vi "Periodic Tasks.vi"(8 "error in":errorcluster) -> ()   [LabVIEW 2016]
doc: "This VI runs in parallel to other robot code. It can contain as many user-defined periodic loops as you need. These can carry out PID or other sorts of timed response."
uses:
  <vilib>/Rock Robotics/WPI/ThirdParty/CanMotor/TalonSRX/WPI_CANTalonSRX_APIControlMode.ctl
  <vilib>/Rock Robotics/WPI/Utilities/WPI_GetSetVariantRefNum.vi
  Robot Global Data.vi
  <vilib>/Rock Robotics/Network Tables/NT Write Boolean.vi
  <vilib>/Rock Robotics/Network Tables/NT Write Number.vi
  <vilib>/Rock Robotics/Network Tables/NT Write Numeric Array.vi
panel:
  out "R3 Latch Shooter":bool
  out "LIDAR Dist IN":dbl
  out "Shooter Speed Increment":dbl=2000.0 format="%#_13g"
  out "LIDAR Dist CM":u16
  # "Gear Catcher forwards, Encoder 1 = +4096\n  Gear Catcher forwards, Encoder 1 = -4096"
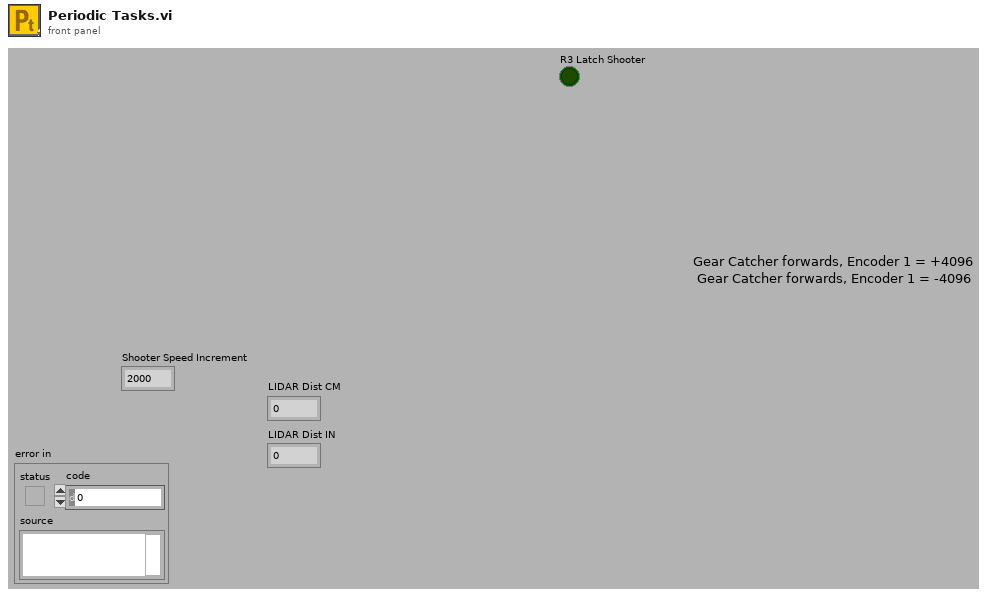
[diagram p1: front panel]
types:
  T1 = typedef "WPI_JoystickDevRef.ctl" = cluster{"Device":T2}
  T2 = typedef "WPI_JoystickDeviceEnum.ctl" = enum16{"USB 0", "USB 1", "USB 2", "USB 3", "USB 4", "USB 5"}
  T3 = typedef "WPI_I2CDevRef.ctl" = cluster{"DevStatus":errorcluster, "Device Address":u8, "Handle":i32, "I2C Bus":T4}
  T4 = typedef "i2c_bus.ctl" = enum16{"I2C On-Board", "I2C MXP", "Invalid"}
  T5 = typedef "WPI_MotorControlDeviceRef.ctl" = cluster{"DeviceStatus":errorcluster, "Type":T6, "PWM":cluster{"PWM Channel":T7, "DeadBand":T8}, "CAN":cluster{"Device Number":u8, "SetOutput VI Ref":variant, "GetOutput VI Ref":variant, "Enable VI Ref":variant, "Disable VI Ref":variant, "Data":variant}, "Invert":bool}
  T6 = typedef "WPI_MotorControlType.ctl" = enum16{"PWM", "CAN"}
  T7 = typedef "FPGA_DIOPWMChannel.ctl" = enum8{"PWM 0", "PWM 1", "PWM 2", "PWM 3", "PWM 4", "PWM 5", "PWM 6", "PWM 7", "PWM 8", "PWM 9", "PWM MXP 0", "PWM MXP 1", "PWM MXP 2", "PWM MXP 3", "PWM MXP 4", "PWM MXP 5", "PWM MXP 6", "PWM MXP 7", "PWM MXP 8", "PWM MXP 9", "Invalid"}
  T8 = typedef "WPI_PWMDeadband.ctl" = cluster{"Name":string, "maxPositivePwm":i32, "minPositivePwm":i32, "centerPwm":i32, "maxNegativePwm":i32, "minNegativePwm":i32, "angularRange":u16}
  T9 = typedef "WPI_CANTalonSRX_APIControlMode.ctl" = enum8{"Percent VBus", "Speed", "Position", "Slave", "Unchanged / Invalid", "Voltage Compensation", "Current", "Motion Profile", "Motion Magic"}
  T10 = typedef "WPI_CANTalonSRX_GlobalStatus.ctl" = cluster{"Applied Throttle":dbl, "Module Enabled":bool, "CAN Error":errorcluster, "Closed Loop Error":dbl, "Forward Limit Switch Closed":bool, "Reverse Limit Switch Closed":bool, "Sensor Position":dbl, "Sensor Velocity":dbl, "Current":dbl, "Sticky Fault - Over Temp":bool, "Sticky Fault - Under Voltage":bool, "Sticky Fault - Forward Limit":bool, "Sticky Fault - Reverse Limit":bool, "Sticky Fault - Forward Soft Limit":bool, "Sticky Fault - Reverse Soft Limit":bool, "Brake is Enabled":bool, "Encoder Position":dbl, "Encoder Velocity":dbl, "Encoder Index Count":dbl, "Encoder A Pin State":bool, "Encoder B Pin State":bool, "Encoder Index Pin State":bool, "Analog In":dbl, "Analog In Velocity":dbl, "Temperature (C)":dbl, "Battery Voltage":dbl, "Control 5 Is Supported":bool, "Current Profile Slot Select":dbl, "Pos Div 8":bool, "Vel Div 4":bool, "Pulse Width Position":i32, "Pulse Width Velocity":i32, "Pulse Width Rise To Rise (us)":i32, "Pulse Width Rise To Fall (us)":i32, "Mot Prof Active Is Under Run":bool, "Mot Prof Active Has Under Run":bool, "Mot Prof Active Is Last":bool, "Mot Prof Active Velocity Only":bool, "Mot Prof Active Is Valid":bool, "Mot Prof Buffer Is Full":bool, "Mot Prof Active Profile Slot Select":i32, "Mot Prof NextID":i32, "Mot Prof Count":i32, "Mot Prof Active Velocity":dbl, "Mot Prof Active Position":dbl, "Mot Prof Output Enable":i32}
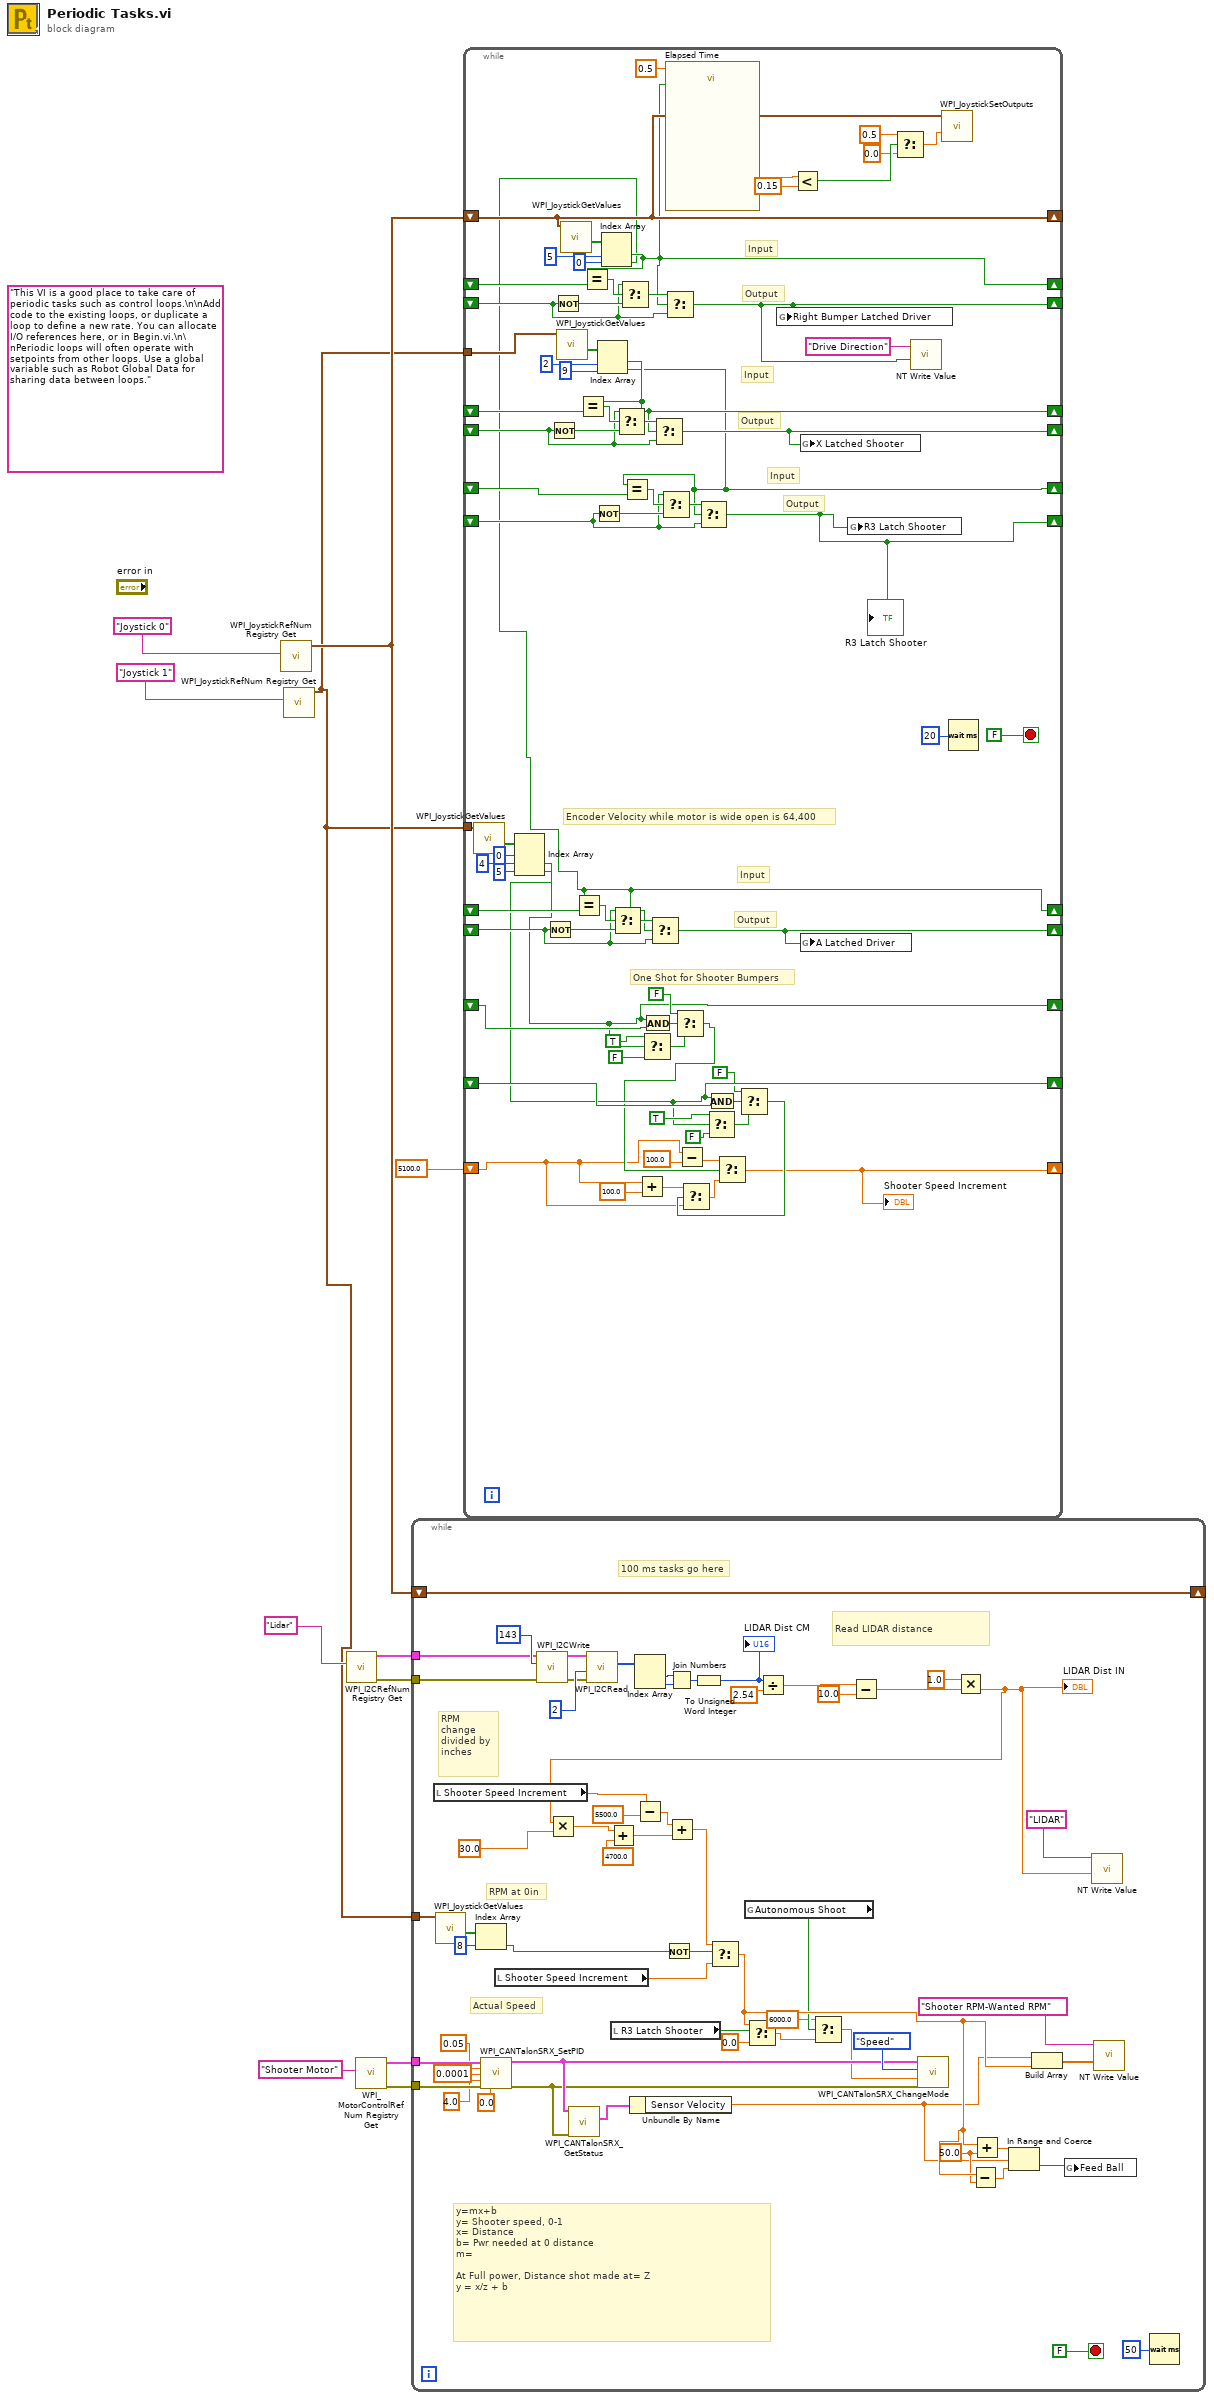
[diagram p0: block diagram]
diagram:
  (unwired) "This VI is a good place to take care of periodic tasks such as control loops.\n\nAdd code to the existing loops, or duplicate a loop to define a new rate. You can allocate I/O references here, or in Begin.vi.\n\nPeriodic loops will often operate with setpoints from other loops. Use a global variable such as Robot Global Data for sharing data between loops."
  n1 = call <vilib>:"WPI_JoystickRefNum Registry Get.vi"("refnum name"="Joystick 0") -> ("JoystickDevRef"=w10:T1)  [unwired: 1 in, 9 out]
  n2 = call <vilib>:"WPI_JoystickRefNum Registry Get.vi"("refnum name"="Joystick 1") -> ("JoystickDevRef"=w1:T1)  [unwired: 1 in, 9 out]
  n3 = call <vilib>:"WPI_I2CRefNum Registry Get.vi"("refnum name"="Lidar") -> ("error out"=w5:errorcluster, "I2CDevRef"=w7:T3)  [unwired: 9 in]
  n4 = call <vilib>:"WPI_MotorControlRefNum Registry Get.vi"("refnum name"="Shooter Motor") -> ("error out"=w2:errorcluster, "MotorControlDevRef"=w3:T5)  [unwired: 9 in]
  n5 = while {
    shift-right: [w68] -> _
    shift-left: w10 -> [w68]
    tunnel: w7 -> [w59]
    tunnel: w5 -> [w55]
    tunnel: w3 -> [w50]
    tunnel: w2 -> [w49]
    tunnel: w1 -> [w13]
    stop <- FALSE stop-if-true
    w32 = 50.0 ("y")
    # "RPM at 0in"
    # "RPM change divided by inches"
    # "y=mx+b\ny= Shooter speed, 0-1\nx= Distance\nb= Pwr needed at 0 distance\nm= \n\nAt Full power, Distance shot made at= Z\ny = x/z + b"
    # "Actual Speed"
    # "Read LIDAR distance"
    # "100 ms tasks go here"
    n6 = local read "Shooter Speed Increment"() -> (w18:dbl)
    n7 = call <vilib>:"WPI_JoystickGetValues.vi"("JoystickDevRef"=w13) -> ("Buttons"=w14:bool[])  [unwired: 6 in, 4 out]
    n8 = Index Array(array=w14, index=8) -> (element=w12:bool)
    n9 = call <vilib>:"WPI_CANTalonSRX_SetPID.vi"("CAN Talon SRX Ref"=w50, "P"=0.05, "I"=0.0001, "D"=4.0, "error in (no error)"=w49, "F"=0.0) -> ("CAN Talon SRX Ref"=w41:T5, "error out"=w40:errorcluster)  [unwired: 8 in]
    n10 = local read "Shooter Speed Increment"() -> (w36:dbl)
    n11 = call <vilib>:"WPI_I2CWrite.vi"("error in (no error)"=w55, "I2CRegister"=u8 143 ("Device Address"), "I2CDevRef"=w59) -> ("error out"=w60:errorcluster, "I2CDevRef"=w61:T3)  [unwired: 7 in]
    n12 = call <vilib>:"WPI_CANTalonSRX_GetStatus.vi"("error in (no error)"=w40, "CAN Talon SRX Ref"=w41) -> ("Talon SRX Status"=w39:T10)  [unwired: 7 in, 2 out]
    n13 = call <vilib>:"WPI_I2CRead.vi"("error in (no error)"=w60, "I2CBytesToRead"=u8 2, "I2CDevRef"=w61) -> ("Data Out"=w67:u8[])  [unwired: 6 in, 2 out]
    n14 = local read "R3 Latch Shooter"() -> (w43:bool)
    n15 = Unbundle By Name(w39) -> ("Sensor Velocity"=w22:dbl)
    n16 = Index Array(array=w67) -> (element #1=w66:u8, element #2=w65:u8)  [unwired: 2 in]
    n17 = Subtract(x=w18, y=5500.0) -> (x-y=w19:dbl)
    n18 = Not(x=w12) -> (.not. x?=w16:bool)
    n19 = Join Numbers(hi=w66, lo=w65) -> ((hi.lo)=w64:u16)
    n20 = To Unsigned Word Integer(number=w64) -> (unsigned 16bit integer=w58:u16)
    "LIDAR Dist CM" <- w58
    n21 = global read "Robot Global Data.vi" "Autonomous Shoot"() -> (w26:bool)
    n22 = Divide(x=w58, y=2.54) -> (x/y=w57:dbl)
    n23 = Subtract(x=w57, y=10.0) -> (x-y=w54:dbl)
    n24 = Multiply(x=1.0, y=w54) -> (x*y=w23:dbl)
    "LIDAR Dist IN" <- w23
    n25 = Multiply(x=w23, y=30.0 ("RPM change/ Inches")) -> (x*y=w30:dbl)
    n26 = Add(x=w30, y=4700.0 ("RPM at 0 in")) -> (x+y=w21:dbl)
    n27 = Add(x=w19, y=w21) -> (x+y=w20:dbl)
    n28 = Select(t=w20, s=w16, f=w36) -> (s? t:f=w33:dbl)
    n29 = Select(t=w33, s=w43, f=0.0) -> (s? t:f=w28:dbl)
    n30 = Select(t=6000.0, s=w26, f=w28) -> (s? t:f=w27:dbl)
    n31 = call <vilib>:"WPI_CANTalonSRX_ChangeMode.vi"("error in (no error)"=w40, "Output"=w27, "Control Mode"=WPI_CANTalonSRX_APIControlMode."Speed", "CAN Talon SRX Ref"=w41) -> ()  [unwired: 6 in, 2 out]
    n32 = Subtract(x=w33, y=w32) -> (x-y=w34:dbl)
    n33 = Add(x=w33, y=w32) -> (x+y=w35:dbl)
    n34 = In Range and Coerce(upper limit=w35, x=w22, lower limit=w34) -> (In Range?=w31:bool)  [unwired: 1 out]
    n35 = Build Array(w22, w33) -> (w38:dbl[])
    n36 = global write "Robot Global Data.vi" "Feed Ball"(w31) -> ()
    n37 = call-poly <vilib>:"NT Write Value.vi"("Numeric"=w23, "Name"="LIDAR") -> ()  [unwired: 9 in, 1 out]
    n38 = call-poly <vilib>:"NT Write Value.vi"("Numeric Array"=w38, "Name"="Shooter RPM-Wanted RPM") -> ()  [unwired: 9 in, 1 out]
    n39 = Wait (ms)(milliseconds to wait=u32 50) -> ()  [unwired: 1 out]
  }
  n40 = while {
    shift-right: [w117] -> _
    shift-left: w10 -> [w117]
    shift-right: [w115] -> _
    shift-left: _ -> [w139]
    shift-right: [w71] -> _
    shift-left: _ -> [w136]
    tunnel: w1 -> [w130]
    shift-right: [w129] -> _
    shift-left: _ -> [w126]
    shift-right: [w128] -> _
    shift-left: _ -> [w127]
    shift-right: [w119] -> _
    shift-left: _ -> [w121]
    shift-right: [w118] -> _
    shift-left: _ -> [w122]
    shift-right: [w73] -> _
    shift-left: _ -> [w105]
    shift-right: [w103] -> _
    shift-left: _ -> [w104]
    tunnel: w1 -> [w100]
    shift-right: [w93] -> _
    shift-left: _ -> [w96]
    shift-right: [w85] -> _
    shift-left: _ -> [w86]
    shift-right: [w77] -> _
    shift-left: 5100.0 -> [w76]
    stop <- FALSE stop-if-true
    # "One Shot for Shooter Bumpers"
    # "Encoder Velocity while motor is wide open is 64,400"
    # "Output"
    # "Input"
    # "Output"
    # "Input"
    # "Output"
    # "Input"
    # "Output"
    # "Input"
    n41 = call <vilib>:"WPI_JoystickGetValues.vi"("JoystickDevRef"=w100) -> ("Buttons"=w101:bool[])  [unwired: 6 in, 4 out]
    n42 = Index Array(array=w101, index #1=0 ("index"), index #2=4 ("index"), index #3=5 ("index")) -> (element #2=w93:bool, element #3=w85:bool)  [unwired: 1 out]
    n43 = Not(x=w104) -> (.not. x?=w106:bool)
    n44 = Not(x=w127) -> (.not. x?=w131:bool)
    n45 = Not(x=w136) -> (.not. x?=w137:bool)
    n46 = call <vilib>:"WPI_JoystickGetValues.vi"("JoystickDevRef"=w130) -> ("Buttons"=w135:bool[])  [unwired: 6 in, 4 out]
    n47 = call <vilib>:"WPI_JoystickGetValues.vi"("JoystickDevRef"=w117) -> ("Buttons"=w142:bool[])  [unwired: 6 in, 4 out]
    n48 = Not(x=w122) -> (.not. x?=w123:bool)
    n49 = Index Array(array=w135, index #1=2 ("index"), index #2=9 ("index")) -> (element #1=w129:bool, element #2=w119:bool)
    n50 = Equal?(x=w129, y=w126) -> (x = y?=w133:bool)
    n51 = Index Array(array=w142, index #1=5 ("index"), index #2=0 ("index")) -> (element #1=w115:bool, element #2=w73:bool)
    n52 = Equal?(x=w73, y=w105) -> (x = y?=w108:bool)
    n53 = Equal?(x=w115, y=w139) -> (x = y?=w140:bool)
    n54 = Select(t=w104, s=w108, f=w106) -> (s? t:f=w107:bool)
    n55 = Select(t=w127, s=w133, f=w131) -> (s? t:f=w132:bool)
    n56 = Select(t=w136, s=w140, f=w137) -> (s? t:f=w138:bool)
    n57 = Equal?(x=w119, y=w121) -> (x = y?=w125:bool)
    n58 = Add(x=w76, y=100.0) -> (x+y=w80:dbl)
    n59 = Select(t=TRUE, s=w93, f=FALSE) -> (s? t:f=w94:bool)
    n60 = And(x=w93, y=w96) -> (x .and. y?=w97:bool)
    n61 = Select(t=w107, s=w73, f=w104) -> (s? t:f=w103:bool)
    n62 = Select(t=w132, s=w129, f=w127) -> (s? t:f=w128:bool)
    n63 = Select(t=w122, s=w125, f=w123) -> (s? t:f=w124:bool)
    n64 = Select(t=w138, s=w115, f=w136) -> (s? t:f=w71:bool)
    n65 = call "Elapsed Time"("Time Target (s)"=0.5, "Reset"=w115) -> ("Elapsed Time (s)"=w114:dbl)  [unwired: 10 in, 7 out]
    n66 = Select(t=FALSE, s=w97, f=w94) -> (s? t:f=w83:bool)
    n67 = Subtract(x=w76, y=100.0 ("x")) -> (x-y=w82:dbl)
    n68 = Select(t=w124, s=w119, f=w122) -> (s? t:f=w118:bool)
    "R3 Latch Shooter" <- w118
    n69 = Select(t=TRUE, s=w85, f=FALSE) -> (s? t:f=w89:bool)
    n70 = And(x=w85, y=w86) -> (x .and. y?=w90:bool)
    n71 = Select(t=FALSE, s=w90, f=w89) -> (s? t:f=w79:bool)
    n72 = Select(t=w80, s=w79, f=w76) -> (s? t:f=w81:dbl)
    n73 = Select(t=w82, s=w83, f=w81) -> (s? t:f=w77:dbl)
    "Shooter Speed Increment" <- w77
    n74 = global write "Robot Global Data.vi" "Right Bumper Latched Driver"(w71) -> ()
    n75 = Less?(x=w114, y=0.15) -> (x < y?=w112:bool)
    n76 = global write "Robot Global Data.vi" "X Latched Shooter"(w128) -> ()
    n77 = global write "Robot Global Data.vi" "A Latched Driver"(w103) -> ()
    n78 = global write "Robot Global Data.vi" "R3 Latch Shooter"(w118) -> ()
    n79 = Select(t=0.5, s=w112, f=0.0) -> (s? t:f=w109:dbl)
    n80 = call-poly <vilib>:"NT Write Value.vi"("Boolean"=w71, "Name"="Drive Direction") -> ()  [unwired: 9 in, 1 out]
    n81 = call <vilib>:"WPI_JoystickSetOutputs.vi"("Right Rumble"=w109, "JoystickDevRef"=w117) -> ()  [unwired: 8 in, 2 out]
    n82 = Wait (ms)(milliseconds to wait=u32 20) -> ()  [unwired: 1 out]
  }
